vi "Demo Navigation Bar.vi"(8 "error in (no error)":errorcluster) -> (0 "error out":errorcluster)   [LabVIEW 2011]
uses:
  VIremote.llb/VIremoteEvent.ctl
  VIremote.llb/VIremoteBarButton.ctl
  VIremote.llb/VIremoteFunction.ctl
  VIremote.llb/VIremoteNavigationBar.ctl
panel:
  in  "More Button":T1
  in  "VIremoteEvent":T2=enum."Connection Closed"
  # "The arrows will point to the wrong places on iPad"
  # "Back button\nwill have a default text that is the same as the previous Top VIs Navigation bar title. The back button text can be set programatically. You can also hide it."
  # "Navigation bar title \nwill have a default text that is the same as the VIs window title.  Can also be set programatically but it should be avoided."
  # "Custom buttons\nYou can add buttons from the left and right side. The ones from the left will appear to the right of the back button if it is shown. The buttons will be linked via reference to normal LabVIEW buttons. The text will be the same as the Boolean Text.Prior to iOS 5 you can have only one button."
  # "Normally you hide this button"
  # "Navigation bar prompt \nAt the top of the bar you can display a text with a smaller font than the title. When the VI is no longer the top VI the prompt will dissapear. This example will set the prompt again when it becomes the Top VI. \nThe promt will make the bar almost twice as high. If you want your panel to shrink when the prompt is displayed you have to resize it. This is especially imortant for Vis that can scroll horizontally.\nThe bar must be visible before you can set the prompt."
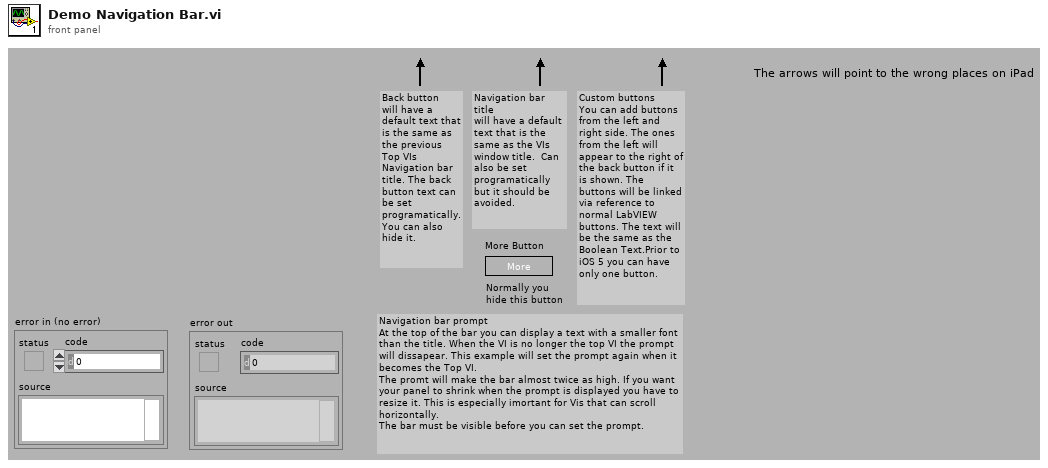
[diagram p1: front panel]
types:
  T1 = typedef "VIremoteBarButton.ctl" = bool
  T2 = typedef "VIremoteEvent.ctl" = enum16{"No Event", "Connection Closed", "Navigate Back", "Enter Background", "Enter Foreground", "Portrait", "Portrait Upside Down", "Landscape Left", "Landscape Right"}
  T3 = typedef "VIremoteNavigationBar.ctl" = enum16{"Show Bar", "Hide Bar", "Clear History", "Set Bar Tint Color", "Set Bar Title", "Set Bar Prompt", "Show Back Button", "Hide Back Button", "Set Back Button Text", "Add Right Button", "Add Left Button", "Remove Button"}
  T4 = typedef "VIremoteFunction.ctl" = enum16{"Do nothing", "Stop controller", "Close this connection", "Show info panel", "Set VI to control", "Set Accelerometer freq (Hz)", "Show Alert message", "Start Sound Input", "Stop Sound Input", "Set Volume (0-100)", "Set sound output Speaker", "Set sound output Receiver", "Play Sound", "Repeat Sound", "Stop Sound", "Pause Sound", "Resume Sound", "Set panel width of caller (320 or 480)", "Set Panel Size to Portrait", "Set Panel Size to Landscape", "Set Panel Size as Current Orientation", "Allow all UI Orientations", "Send user notification", "Disable Scrolling", "Normal Scrolling", "Page Scrolling", "Set Scroll Offset", "Page Indicator Position"}
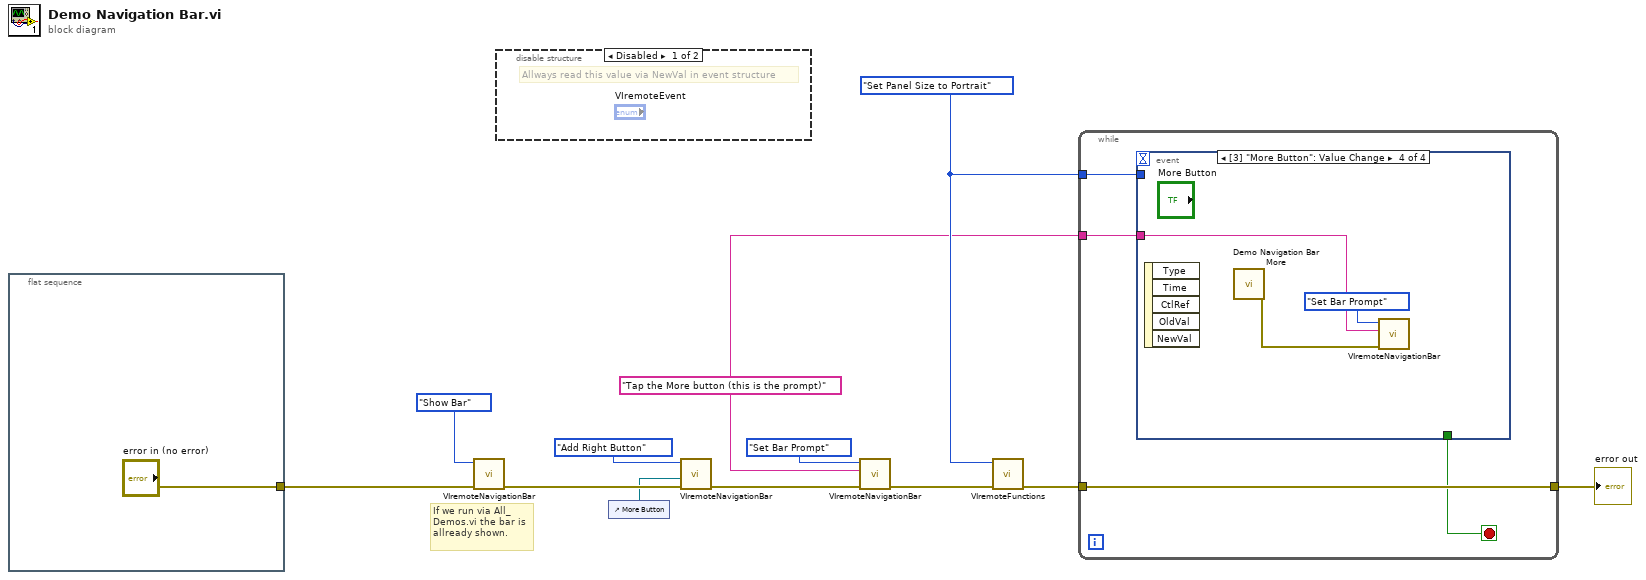
[diagram p0: block diagram]
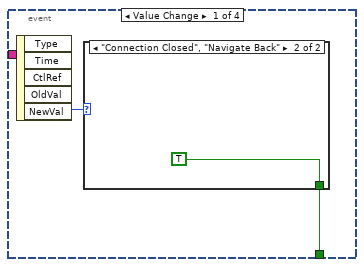
[diagram p3: hidden frame]
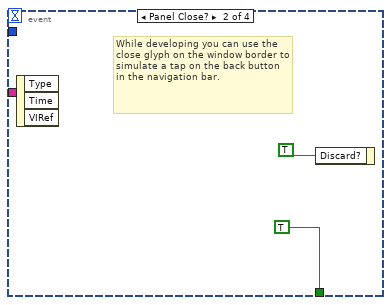
[diagram p5: hidden frame]
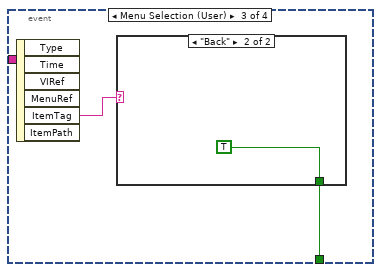
[diagram p6: hidden frame]
diagram:
  w10 = "Tap the More button (this is the prompt)" ("String")
  w12 = VIremoteFunction."Set Panel Size to Portrait" ("Function")
  # "If we run via All_Demos.vi the bar is allready shown."
  n1 = flat-sequence {
    tunnel: ["error in (no error)"] -> w9
    frame #0 {
    }
  }
  n2 = call "VIremoteNavigationBar.vi"("error in (no error)"=w9, "Func"=VIremoteNavigationBar."Show Bar") -> ("error out"=w6:errorcluster)  [unwired: 4 in, 5 out]
  n3 = disable-structure shown="Disabled" {
    frame Disabled {
      # "Allways read this value via NewVal in event structure"
    }
    frame Enabled {
    }
  }
  n4 = control-ref of="More Button"() -> (w4:refnum<vi>)
  n5 = call "VIremoteNavigationBar.vi"("error in (no error)"=w6, "Button reference"=w4, "Func"=VIremoteNavigationBar."Add Right Button") -> ("error out"=w2:errorcluster)  [unwired: 3 in, 5 out]
  n6 = call "VIremoteNavigationBar.vi"("error in (no error)"=w2, "String (\"\")"=w10, "Func"=VIremoteNavigationBar."Set Bar Prompt") -> ("error out"=w11:errorcluster)  [unwired: 3 in, 5 out]
  n7 = call "VIremoteFunctions.vi"("error in (no error)"=w11, "Function"=w12) -> ("error out"=w8:errorcluster)  [unwired: 4 in, 5 out]
  n8 = while {
    tunnel: [w17] -> w1
    tunnel: w8 -> [w17]
    tunnel: w12 -> [w15]
    tunnel: w10 -> [w14]
    stop <- w16 stop-if-true
    n9 = event shown="[3] \"More Button\": Value Change" {
      selector: _ -> [_ _ _ _]
      dyn-events: _ -> [_ _ _ _]
      timeout: _ -> [_ _ _ _]
      tunnel: [w18 TRUE ("Discard?") w23 _] -> w16
      tunnel: w15 -> [_ _ _ _]
      tunnel: w14 -> [_ _ _ w26]
      event Value Change {
        n10 = event-data() -> ("NewVal"=w19:T2)  [unwired: 5 out]
        n11 = case shown="\"Connection Closed\", \"Navigate Back\"" w19 {
          tunnel: [_ TRUE] -> w18
          frame "No Event", Default {
          }
          frame "Connection Closed", "Navigate Back" {
          }
        }
      }
      event Panel Close? {
        # "While developing you can use the close glyph on the window border to simulate a tap on the back button in the navigation bar."
        n12 = event-data() -> ()  [unwired: 4 out]
        n13 = event-data("Discard?"=TRUE) -> ()  [unwired: 1 in, 1 out]
      }
      event Menu Selection (User) {
        n14 = event-data() -> ("ItemTag"=w24:string)  [unwired: 6 out]
        n15 = case shown="\"Back\"" w24 {
          tunnel: [_ TRUE ("Discard?")] -> w23
          frame Default {
          }
          frame "Back" {
          }
        }
      }
      event Value Change {
        n16 = event-data() -> ()  [unwired: 6 out]
        n17 = call "Demo Navigation Bar More.vi"() -> ("error out"=w27:errorcluster)  [unwired: 1 in, 10 out]
        n18 = call "VIremoteNavigationBar.vi"("error in (no error)"=w27, "String (\"\")"=w26, "Func"=VIremoteNavigationBar."Set Bar Prompt") -> ()  [unwired: 2 in, 7 out]
      }
    }
  }
  "error out" <- w1
